vi "APS get sampling data.vi"(7 "Status":i32, 8 "error in (no error)":errorcluster caption="错误输入（无错误）", 9 "DataArr":T1, 10 "Length":i32, 11 "Board_ID":i32) -> (0 "error out":errorcluster caption="错误输出", 1 "DataArr out":T1, 2 "Length out":i32, 3 "function return":i32, 5 "Status out":i32)   [LabVIEW 2011, in "APS168.lvlib"]
doc: "I32 FNTYPE APS_get_sampling_data( I32 Board_ID, I32 *Length, STR_SAMP_DATA_4CH *DataArr, I32 *Status );"
uses:
  APS168.lvlib
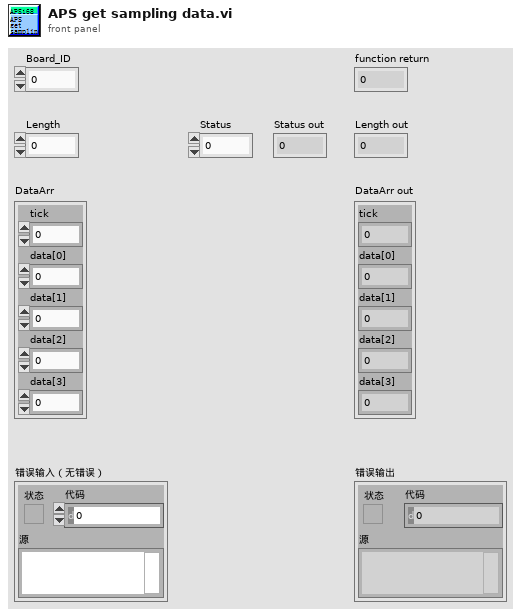
[diagram p1: front panel]
types:
  T1 = cluster{"tick":i32, "data[0]":i32, "data[1]":i32, "data[2]":i32, "data[3]":i32}
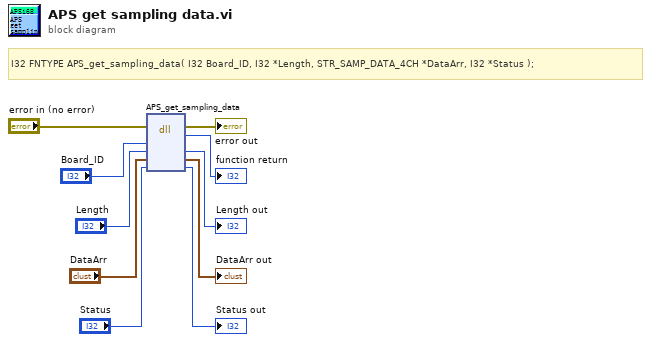
[diagram p0: block diagram]
diagram:
  # "I32 FNTYPE APS_get_sampling_data( I32 Board_ID, I32 *Length, STR_SAMP_DATA_4CH *DataArr, I32 *Status );"
  n1 = dll-call lib="PTH1Labs E软件ADLINK 204CAPS_1_7_1_LIB line 连续运动204APS168.*" fn="APS_get_sampling_data"(error in="error in (no error)", "Board_ID"="Board_ID", "Length"="Length", "DataArr"="DataArr", "Status"="Status") -> (error out=→"error out":errorcluster, →"function return":i32, "Length"=→"Length out":i32, "DataArr"=→"DataArr out":T1, "Status"=→"Status out":i32)  [unwired: 3 in, 1 out]
